vi "Sub Pabel FGV.vi"(7 "Command":enum16{"Set", "Get"}(ring), 8 "error in (no error)":errorcluster, 10 "Sub Panel":refnum<vi>, 11 "Plug in VI":refnum<vi>[](array[refnum])) -> (0 "error out":errorcluster, 2 "Sub Panel":refnum<vi>, 3 "Plug in VI":refnum<vi>[](array[refnum]))   [LabVIEW 2021, in "User Interface.lvlib"]
uses:
  User Interface.lvlib
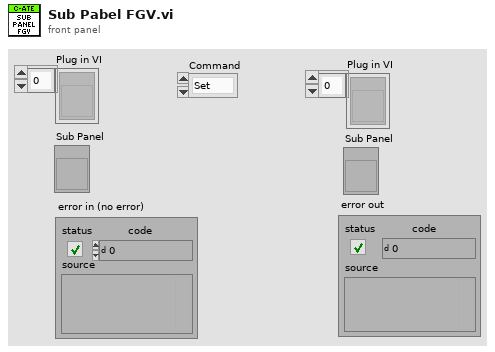
[diagram p1: front panel]
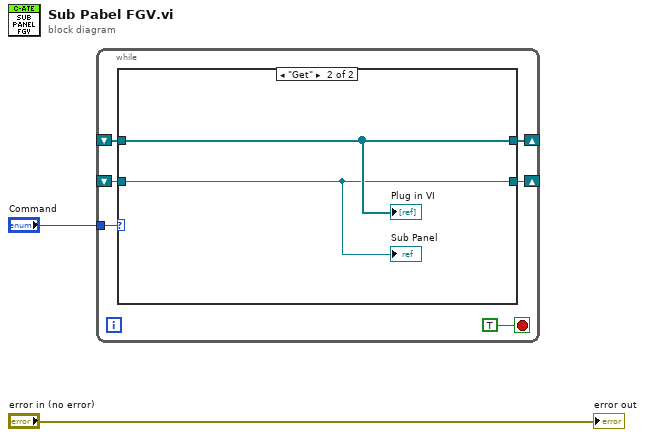
[diagram p0: block diagram]
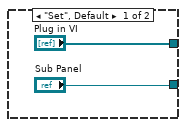
[diagram p2: hidden frame]
diagram:
  n1 = while {
    tunnel: "Command" -> [w7]
    shift-right: [w6] -> _
    shift-left: _ -> [w5]
    shift-right: [w4] -> _
    shift-left: _ -> [w3]
    stop <- TRUE stop-if-true
    n2 = case shown="\"Get\"" w7 {
      tunnel: ["Plug in VI" w12] -> w6
      tunnel: w5 -> [_ w12]
      tunnel: ["Sub Panel" w11] -> w4
      tunnel: w3 -> [_ w11]
      frame "Set", Default {
      }
      frame "Get" {
        "Plug in VI" <- w12
        "Sub Panel" <- w11
      }
    }
  }
  "error out" <- "error in (no error)"
